vi "Get Pixel.vi"(8 "error in (no error)":errorcluster, 9 "y":i32, 10 "x":i32, 11 "senseHatDisplay in":refnum<class "RPI.SenseHat.Display.lvclass">) -> (0 "error out":errorcluster, 2 "Pixel":refnum<class "Pixel.lvclass">, 3 "senseHatDisplay out":refnum<class "RPI.SenseHat.Display.lvclass">)   [LabVIEW 2020, in "RPI.SenseHat.Display.lvlib" / "RPI.SenseHat.Display.lvclass"]
uses:
  RPI.SenseHat.Display.lvclass
  Pixel/Pixel.lvclass
  RPI.SenseHat.Display.lvclass/RPI.SenseHat.Display.ctl
  Image/Image.lvclass
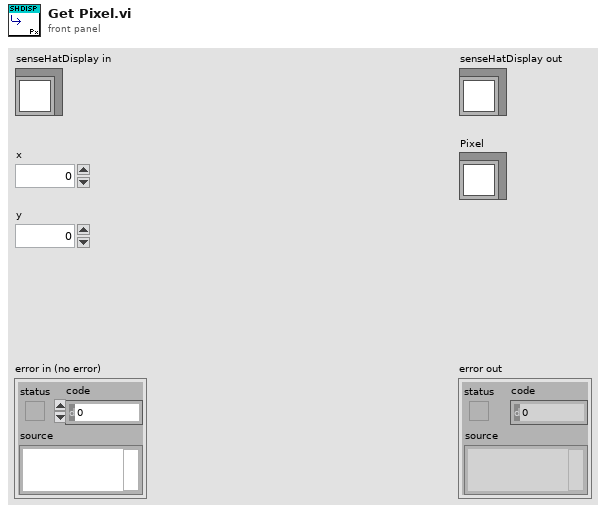
[diagram p1: front panel]
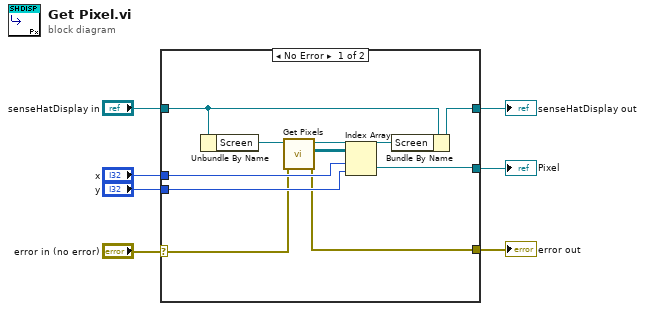
[diagram p0: block diagram]
diagram:
  n1 = case shown="No Error" "error in (no error)" {
    selector: "error in (no error)" -> [w10 w19]
    tunnel: [w9 w19] -> w6
    tunnel: [w12 w18] -> w4
    tunnel: "senseHatDisplay in" -> [w17 w18]
    tunnel: "x" -> [w14 _]
    tunnel: "y" -> [w13 _]
    tunnel: [w8 _] -> w1
    frame No Error {
      n2 = Unbundle By Name(w17) -> ("Screen"=w16:refnum<class "Image.lvclass">)
      n3 = call "Get Pixels.vi"("error in (no error)"=w10, "Image in"=w16) -> ("error out"=w9:errorcluster, "Pixels"=w15:refnum<class "Pixel.lvclass">[][], "Image out"=w11:refnum<class "Image.lvclass">)  [unwired: 7 in]
      n4 = Index Array(array=w15, index (row)=w14, index (col)=w13) -> (element=w8:refnum<class "Pixel.lvclass">)
      n5 = Bundle By Name(cluster=w17, "Screen"=w11) -> (w12:refnum<class "RPI.SenseHat.Display.lvclass">)
    }
    frame Error {
    }
  }
  "error out" <- w6
  "senseHatDisplay out" <- w4
  "Pixel" <- w1
